vi "Get_command_string_from_multipart_message.vi"(0 "Multipart message in":string[](array[string]), 11 "error in (no error)":errorcluster) -> (4 "command string out":string, 15 "error out":errorcluster)   [LabVIEW 2019, in "mmW_commands.lvlib"]
uses:
  mmW_commands.lvlib
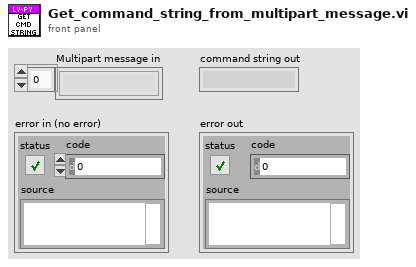
[diagram p1: front panel]
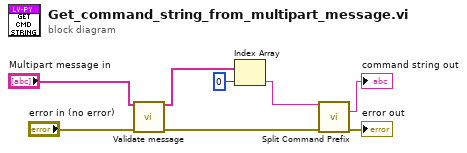
[diagram p0: block diagram]
diagram:
  n1 = call "Validate message.vi"("multipart message in"="Multipart message in", "error in (no error)"="error in (no error)") -> ("multipart message out"=w3:string[], "error out"=w6:errorcluster)  [unwired: 8 in, 4 out]
  n2 = Index Array(array=w3, index=0) -> (element=w1:string)
  n3 = call "Split Command Prefix.vi"("command string in"=w1, "error in"=w6) -> ("command out"=→"command string out":string, "error out"=→"error out":errorcluster)  [unwired: 11 in, 1 out]
